vi "19.4-FIR-Wnd-App.vi"() -> ()   [LabVIEW 2020]
doc: "Uses the Median Filter VI to analyze pulses in the presence of noise. The example generates a pulse contaminated with Gaussian noise and applies a median filter. For comparison purposes, the VI computes the pulse parameters of the filtered pulse."
uses:
  <vilib>/Analysis/4window.llb/windowTd.ctl
  <vilib>/Analysis/3filter.llb/Filter Passband Type.ctl
  <vilib>/Analysis/3filter.llb/FIR Windowed Filter (DBL).vi
  <vilib>/Analysis/NI_AALBase.lvlib
  <vilib>/Analysis/NI_AALPro.lvlib
panel:
  in  "window":T1=5 items=["Rectangle"=0, "Hanning"=1, "Hamming"=2, "Blackman-Harris"=3, "Exact Blackman"=4, "Blackman"=5, "Flat Top"=6, "4 Term B-Harris "=7, "7 Term B-Harris"=8, "Low Sidelobe"=9, "Blackman Nuttall"=11, "Triangle"=30, "Bartlett-Hanning"=31, "Bohman"=32, "Parzen"=33, "Welch"=34, "Kaiser"=60, "Dolph-Chebyshev"=61, "Gaussian"=62]
  out "x[n]-filtered":dbl[](graph)
  out "X[k]-Filtered":dbl[](graph)
  out "X[k]":dbl[](graph)
  out "x[n]":dbl[](graph)
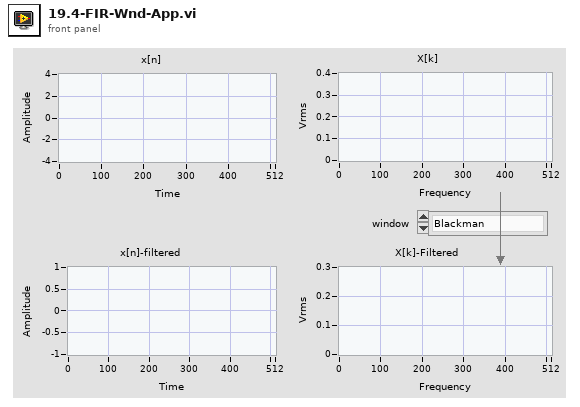
[diagram p1: front panel]
types:
  T1 = typedef "NI_AALPro.lvlib/windowTd.ctl" = u32
  T2 = typedef "NI_AALBase.lvlib/Filter Passband Type.ctl" = enum32{"Lowpass", "Highpass", "Bandpass", "Bandstop"}
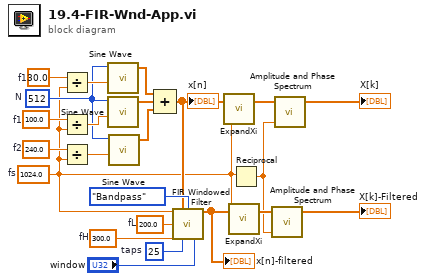
[diagram p0: block diagram]
diagram:
  w10 = 30.0  # f1
  w14 = 25  # taps
  w16 = 300.0  # fH
  w17 = 200.0  # fL
  w2 = 1024.0  # fs
  w21 = 240.0  # f2
  w23 = 100.0  # f1
  w8 = 512  # N
  n1 = Divide(x=w10, y=w2) -> (x/y=w9:dbl)
  n2 = Divide(x=w23, y=w2) -> (x/y=w22:dbl)
  n3 = Divide(x=w21, y=w2) -> (x/y=w20:dbl)
  n4 = call <vilib>:"Sine Wave.vi"("samples"=w8, "frequency"=w9) -> ("sine wave"=w7:dbl[])  [unwired: 3 in, 2 out]
  n5 = call <vilib>:"Sine Wave.vi"("samples"=w8, "frequency"=w22) -> ("sine wave"=w19:dbl[])  [unwired: 3 in, 2 out]
  n6 = call <vilib>:"Sine Wave.vi"("samples"=w8, "frequency"=w20) -> ("sine wave"=w18:dbl[])  [unwired: 3 in, 2 out]
  n7 = Compound Arithmetic op=ADD(w7, w19, w18) -> (w12:dbl[])
  "x[n]" <- w12
  n8 = call-poly <vilib>:"FIR Windowed Filter.vi"("sampling freq: fs"=w2, "X"=w12, "filter type"=Filter_Passband_Type."Bandpass", "low cutoff freq: fl"=w17, "high cutoff freq: fh"=w16, "taps"=w14, "window"="window") -> ("Filtered X"=w11:dbl[])  [unwired: 7 in, 1 out]
  "x[n]-filtered" <- w11
  n9 = call "ExpandXi.vi"("N"=w2, "X"=w12) -> ("X 2"=w5:dbl[])  [unwired: 1 in]
  n10 = call "ExpandXi.vi"("N"=w2, "X"=w11) -> ("X 2"=w4:dbl[])  [unwired: 1 in]
  n11 = Reciprocal(x=w2) -> (1/x=w1:dbl)
  n12 = call <vilib>:"Amplitude and Phase Spectrum.vi"("dt"=w1, "Signal (V)"=w4) -> ("Amp Spectrum Mag (Vrms)"=→"X[k]-Filtered":dbl[])  [unwired: 1 in, 2 out]
  n13 = call <vilib>:"Amplitude and Phase Spectrum.vi"("dt"=w1, "Signal (V)"=w5) -> ("Amp Spectrum Mag (Vrms)"=→"X[k]":dbl[])  [unwired: 1 in, 2 out]
